vi "NanotecSMCPD.position in range for safety function.vi"(0 "i ref in":refnum<vi>, 2 "axisIndex":i32, 3 "reqPosition":dbl, 4 "absolute":bool, 5 "error in (no error)":errorcluster) -> (14 "i ref out":refnum<vi>, 16 "in range":bool, 19 "error out":errorcluster)   [LabVIEW 2014, in "NanotecSMCPD.lvlib"]
doc: "Checks, if the requested position is in range."
uses:
  NanotecSMCPD.lvlib
  CSCore/CSApplicationBaseClasses/MotorBase/MotorBase.lvlib
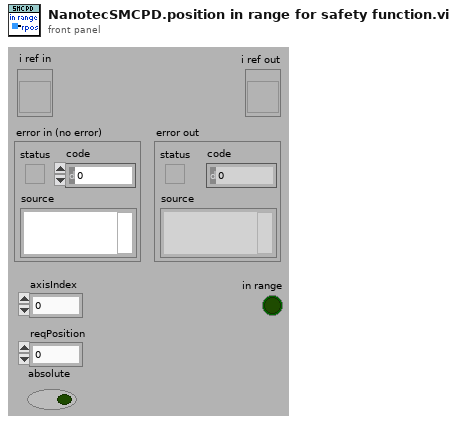
[diagram p1: front panel]
types:
  T1 = typedef "MotorBase.lvlib/MotorBase.i attribute.ctl" = cluster{"defaultAxisIndex":i32, "logicalName":string[], "nOfAxes":i32, "physicalName":string[], "scaling":dbl[], "units":string[], "defaulAxisIndexID":i32, "logicalNameID":i32, "nOfAxesID":i32, "physicalNameID":i32, "unitID":i32, "actValues":T2, "nomValues":T2}
  T2 = typedef "MotorBase.lvlib/MotorBase.parameters.ctl" = cluster{"services":cluster{"onOff":bool[], "startVelocity":dbl[], "stopVelocity":dbl[], "acceleration":dbl[], "rangeMin":dbl[], "rangeMax":dbl[], "status":T3[], "position":dbl[]}, "serviceIDs":cluster{"onOffID":i32, "startVelocityID":i32, "stopVelocityID":i32, "accelerationID":i32, "rangeMinID":i32, "rangeMaxID":i32, "statusID":i32, "positionID":i32}}
  T3 = typedef "MotorBase.lvlib/MotorBase.statusType.ctl" = u32
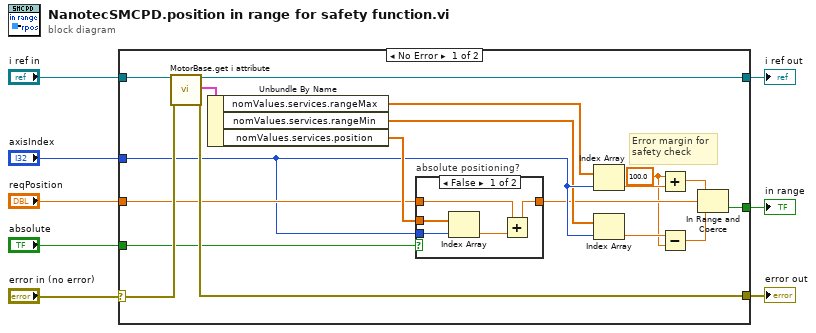
[diagram p0: block diagram]
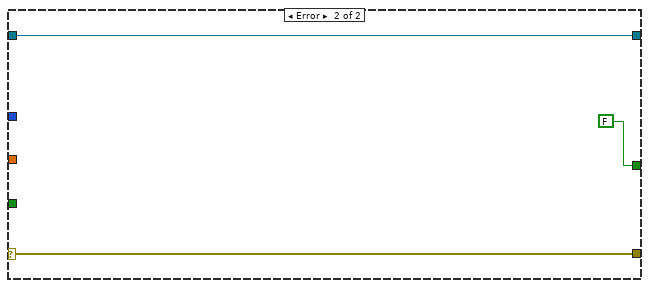
[diagram p3: hidden frame]
diagram:
  n1 = case shown="No Error" "error in (no error)" {
    selector: "error in (no error)" -> [w25 w34]
    tunnel: "i ref in" -> [w26 w35]
    tunnel: [w24 w34] -> w6
    tunnel: [w23 w35] -> w5
    tunnel: [w14 FALSE] -> w4
    tunnel: "axisIndex" -> [w18 _]
    tunnel: "absolute" -> [w21 _]
    tunnel: "reqPosition" -> [w19 _]
    frame No Error {
      w9 = 100.0 ("x")
      # "Error margin for\nsafety check"
      n2 = call "MotorBase.get i attribute.vi"("i ref in"=w26, "error in (no error)"=w25) -> ("i ref out"=w23:refnum<vi>, "i attribute"=w22:T1, "error out"=w24:errorcluster)  [unwired: 15 in]
      n3 = Unbundle By Name(w22) -> ("nomValues.services.rangeMax"=w17:dbl[], "nomValues.services.rangeMin"=w16:dbl[], "nomValues.services.position"=w20:dbl[])
      n4 = case "absolute positioning?" shown="False" w21 {
        tunnel: w20 -> [w31 _]
        tunnel: w18 -> [w30 _]
        tunnel: w19 -> [w28 w32]
        tunnel: [w27 w32] -> w15
        frame False {
          n5 = Index Array(array=w31, index=w30) -> (element=w29:dbl)
          n6 = Add(x=w28, y=w29) -> (x+y=w27:dbl)
        }
        frame True {
        }
      }
      n7 = Index Array(array=w17, index=w18) -> (element=w13:dbl)
      n8 = Index Array(array=w16, index=w18) -> (element=w10:dbl)
      n9 = Add(x=w9, y=w13) -> (x+y=w12:dbl)
      n10 = Subtract(x=w10, y=w9) -> (x-y=w11:dbl)
      n11 = In Range and Coerce(upper limit=w12, x=w15, lower limit=w11) -> (In Range?=w14:bool)  [unwired: 1 out]
    }
    frame Error {
    }
  }
  "error out" <- w6
  "i ref out" <- w5
  "in range" <- w4
